vi "dataUnpackI32Array.vi"(8 "errorIn":errorcluster, 11 "data":variant) -> (0 "errorOut":errorcluster, 3 "SGLArray":i32[](array[numeric]))   [LabVIEW 2017]
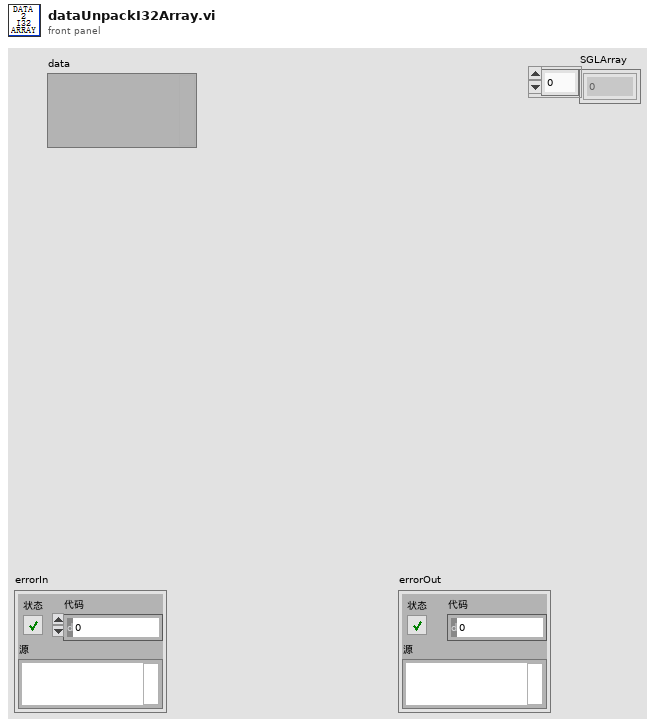
[diagram p1: front panel]
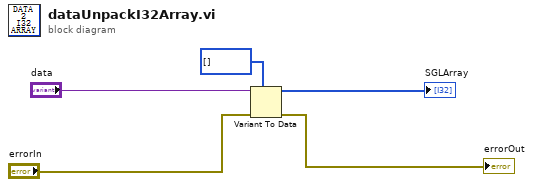
[diagram p0: block diagram]
diagram:
  n1 = Variant To Data(error in="errorIn", type=i32[] [], Variant="data") -> (data=→"SGLArray":i32[], error out=→"errorOut":errorcluster)
